vi "List Firmware Files.vi"(11 "error in (no error)":errorcluster) -> (4 "default firmware path":path, 6 "firmware filenames":string[](array[string]), 15 "error out":errorcluster)   [LabVIEW 2020, in "SLSC.lvlib"]
uses:
  <vilib>/SLSC/SLSC.lvlib
  <vilib>/Utility/sysdir.llb/System Directory Type.ctl
  kernel32.dll
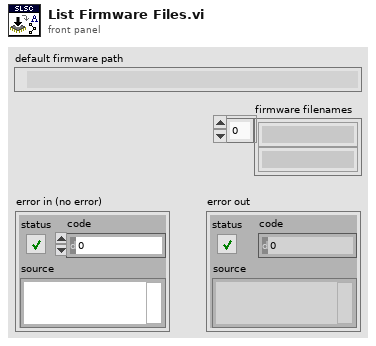
[diagram p1: front panel]
types:
  T1 = typedef "System Directory Type.ctl" = i32
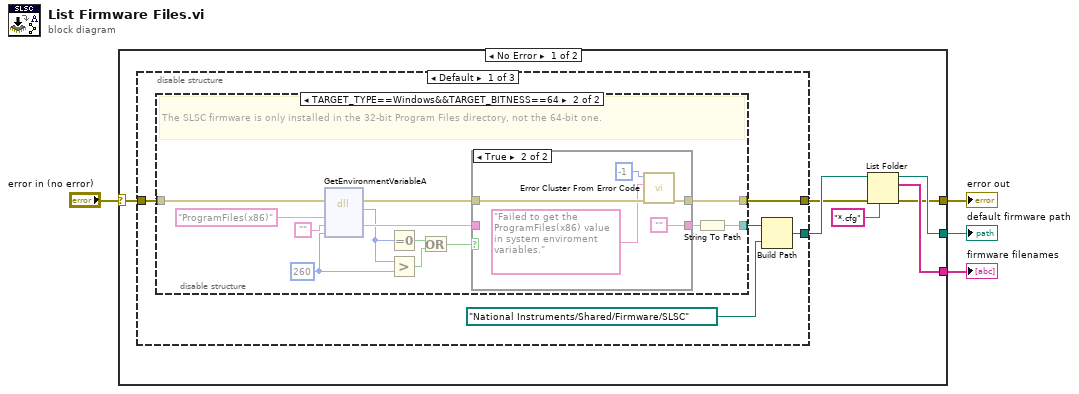
[diagram p0: block diagram]
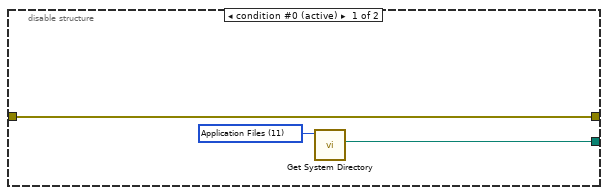
[diagram p2: hidden frame]
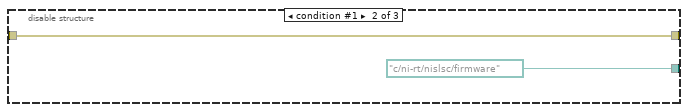
[diagram p4: hidden frame]
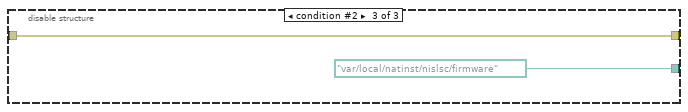
[diagram p5: hidden frame]
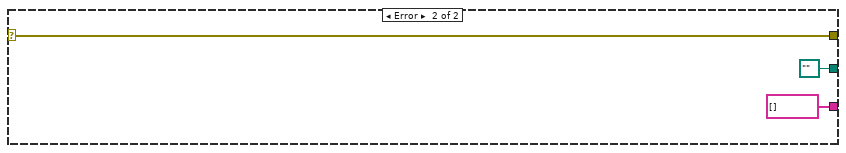
[diagram p6: hidden frame]
diagram:
  n1 = case shown="No Error" "error in (no error)" {
    selector: "error in (no error)" -> [w11 w45]
    tunnel: [w8 path "" ("appended path")] -> w3
    tunnel: [w5 w45] -> w2
    tunnel: [w7 string[] [] ("filenames")] -> w1
    frame No Error {
      n2 = disable-structure shown="Default" {
        disable-tunnel: [w14 path "c:/ni-rt/nislsc/firmware" path "/var/local/natinst/nislsc/firmware"] -> w9
        disable-tunnel: w11 -> [w13 w40 w42]
        disable-tunnel: [w12 w40 w42] -> w6
        frame condition #0 (active) {
          n3 = disable-structure shown="TARGET_TYPE==Windows&&TARGET_BITNESS==64" {
            disable-tunnel: [w18 w21] -> w16
            disable-tunnel: w13 -> [w17 w31]
            disable-tunnel: [w17 w28] -> w12
            frame condition #0 (active) {
              w19 = T1 11 items=["User Home"=0, "User Desktop"=1, "User Documents"=2, "User Application Data"=3, "User Preferences"=4, "User Temporary"=5, "Public Documents"=6, "Public Application Data"=7, "Public Preferences"=8, "Public Cache"=13, "System Core Libraries"=9, "System Installed Libraries"=10, "Application Files"=11, "Boot Volume Root"=12] ("system directory type")
              n4 = call <vilib>:"Get System Directory.vi"("system directory type"=w19) -> ("system directory"=w18:path)  [unwired: 10 in]
            }
            frame condition #1 {
              w25 = u32 260 ("nSize")
              # "The SLSC firmware is only installed in the 32-bit Program Files directory, not the 64-bit one."
              n5 = dll-call lib="kernel32.dll" fn="GetEnvironmentVariableA"(error in=w31, "lpName"="ProgramFiles(x86)", "lpBuffer"="", "nSize"=w25) -> (error out=w29:errorcluster, "return type"=w20:u32, "lpBuffer"=w23:string)  [unwired: 4 in, 1 out]
              n6 = Equal To 0?(x=w20) -> (x = 0?=w27:bool)
              n7 = Greater?(x=w20, y=w25) -> (0:w26:bool)
              n8 = Or(x=w27, y=w26) -> (x .or. y?=w24:bool)
              n9 = case shown="True" w24 {
                tunnel: w29 -> [w34 w39]
                tunnel: [w34 w36] -> w28
                tunnel: w23 -> [w33 _]
                tunnel: [w33 ""] -> w22
                frame False {
                }
                frame True {
                  n10 = call <vilib>:"Error Cluster From Error Code.vi"("error in (no error)"=w39, "error message (\"\")"="Failed to get the ProgramFiles(x86) value in system enviroment variables." ("error message (\"\")"), "error code (0)"=-1) -> ("error out"=w36:errorcluster)  [unwired: 6 in]
                }
              }
              n11 = String To Path(string=w22) -> (path=w21:path)
            }
          }
          n12 = Build Path(base path=w16, name or relative path=path "National Instruments/Shared/Firmware/SLSC") -> (appended path=w14:path)
        }
        frame condition #1 {
        }
        frame condition #2 {
        }
      }
      n13 = List Folder(path=w9, pattern="*.cfg", error in=w6) -> (path out=w8:path, filenames=w7:string[], error out=w5:errorcluster)  [unwired: 1 in, 1 out]
    }
    frame Error {
    }
  }
  "default firmware path" <- w3
  "error out" <- w2
  "firmware filenames" <- w1
